vi "main RT.vi"   [LabVIEW 2024]
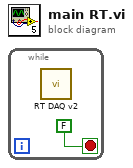
[diagram p0: block diagram]
diagram:
  n1 = while {
    stop <- FALSE stop-if-true
    n2 = call "RT DAQ v2.vi"() -> ()  [unwired: 12 in]
  }
